vi "svfa_Initial Guess for Tone Estimation (magnitude).vi"(8 "FFT size":i32, 9 "window size":i32, 10 "window":T1(ring), 11 "three fingers":cluster{"f0":dbl, "df":dbl, "spectrum":dbl[]}={"f0"=0.0, "df"=1.0, "spectrum"=[]} {"spectrum" format="%.4f"; "df" format="%.4f"; "f0" format="%.4f"}) -> (0 "range":cluster{"f upper":dbl, "f lower":dbl} {"f lower" format="%.2e"; "f upper" format="%.2e"}, 3 "initial guess":dbl format="%.9f")   [LabVIEW 2017]
uses:
  <vilib>/Analysis/4window.llb/windowTd.ctl
  <vilib>/addons/_NISVFA/_Spectrum Processing/subVIs/svfa_Tone Estimation Subroutine G(f) (magnitude).vi
  <vilib>/addons/_NISVFA/_Spectrum Processing/subVIs/svfa_Tone Estimation Subroutine G(f) (first derivative) (magnitude).vi
  <vilib>/Analysis/NI_AALPro.lvlib
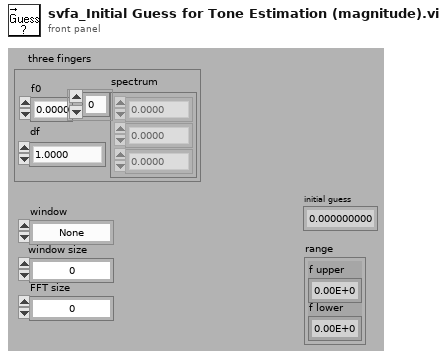
[diagram p1: front panel]
types:
  T1 = enum16{"None ", "Hanning", "Hamming", "Blackman-Harris", "Exact Blackman", "Blackman", "Flat Top", "4 Term B-Harris ", "7 Term B-Harris", "Low Sidelobe"}
  T2 = typedef "NI_AALPro.lvlib/windowTd.ctl" = u32
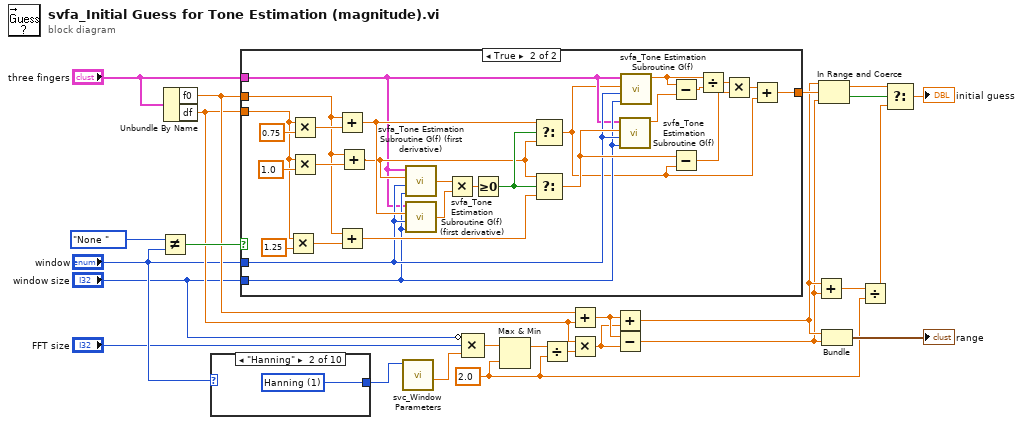
[diagram p0: block diagram]
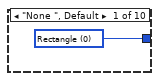
[diagram p2: hidden frame]
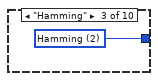
[diagram p3: hidden frame]
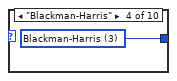
[diagram p4: hidden frame]
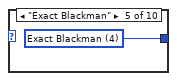
[diagram p5: hidden frame]
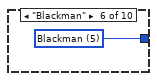
[diagram p6: hidden frame]
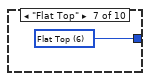
[diagram p7: hidden frame]
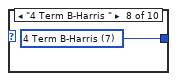
[diagram p8: hidden frame]
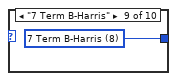
[diagram p9: hidden frame]
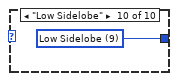
[diagram p10: hidden frame]
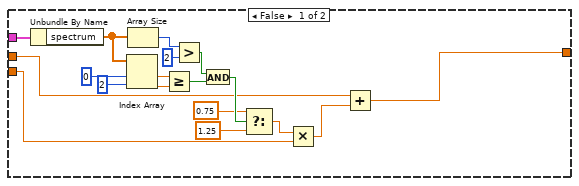
[diagram p11: hidden frame]
diagram:
  w3 = 2.0 ("y")
  n1 = Not Equal?(x=T1."None " ("window"), y="window") -> (x != y?=w23:bool)
  n2 = Unbundle By Name("three fingers") -> ("f0"=w17:dbl, "df"=w14:dbl)
  n3 = case shown="\"Hanning\"" "window" {
    tunnel: [w26 w27 w28 w29 w30 w31 w32 w33 w34 w35] -> w4
    frame "None ", Default {
      w26 = T2 0 items=["Rectangle"=0, "Hanning"=1, "Hamming"=2, "Blackman-Harris"=3, "Exact Blackman"=4, "Blackman"=5, "Flat Top"=6, "4 Term B-Harris "=7, "7 Term B-Harris"=8, "Low Sidelobe"=9, "Blackman Nuttall"=11, "Triangle"=30, "Bartlett-Hanning"=31, "Bohman"=32, "Parzen"=33, "Welch"=34, "Kaiser"=60, "Dolph-Chebyshev"=61, "Gaussian"=62] ("window")
    }
    frame "Hanning" {
      w27 = T2 1 items=["Rectangle"=0, "Hanning"=1, "Hamming"=2, "Blackman-Harris"=3, "Exact Blackman"=4, "Blackman"=5, "Flat Top"=6, "4 Term B-Harris "=7, "7 Term B-Harris"=8, "Low Sidelobe"=9, "Blackman Nuttall"=11, "Triangle"=30, "Bartlett-Hanning"=31, "Bohman"=32, "Parzen"=33, "Welch"=34, "Kaiser"=60, "Dolph-Chebyshev"=61, "Gaussian"=62] ("window")
    }
    frame "Hamming" {
      w28 = T2 2 items=["Rectangle"=0, "Hanning"=1, "Hamming"=2, "Blackman-Harris"=3, "Exact Blackman"=4, "Blackman"=5, "Flat Top"=6, "4 Term B-Harris "=7, "7 Term B-Harris"=8, "Low Sidelobe"=9, "Blackman Nuttall"=11, "Triangle"=30, "Bartlett-Hanning"=31, "Bohman"=32, "Parzen"=33, "Welch"=34, "Kaiser"=60, "Dolph-Chebyshev"=61, "Gaussian"=62] ("window")
    }
    frame "Blackman-Harris" {
      w29 = T2 3 items=["Rectangle"=0, "Hanning"=1, "Hamming"=2, "Blackman-Harris"=3, "Exact Blackman"=4, "Blackman"=5, "Flat Top"=6, "4 Term B-Harris "=7, "7 Term B-Harris"=8, "Low Sidelobe"=9, "Blackman Nuttall"=11, "Triangle"=30, "Bartlett-Hanning"=31, "Bohman"=32, "Parzen"=33, "Welch"=34, "Kaiser"=60, "Dolph-Chebyshev"=61, "Gaussian"=62] ("window")
    }
    frame "Exact Blackman" {
      w30 = T2 4 items=["Rectangle"=0, "Hanning"=1, "Hamming"=2, "Blackman-Harris"=3, "Exact Blackman"=4, "Blackman"=5, "Flat Top"=6, "4 Term B-Harris "=7, "7 Term B-Harris"=8, "Low Sidelobe"=9, "Blackman Nuttall"=11, "Triangle"=30, "Bartlett-Hanning"=31, "Bohman"=32, "Parzen"=33, "Welch"=34, "Kaiser"=60, "Dolph-Chebyshev"=61, "Gaussian"=62] ("window")
    }
    frame "Blackman" {
      w31 = T2 5 items=["Rectangle"=0, "Hanning"=1, "Hamming"=2, "Blackman-Harris"=3, "Exact Blackman"=4, "Blackman"=5, "Flat Top"=6, "4 Term B-Harris "=7, "7 Term B-Harris"=8, "Low Sidelobe"=9, "Blackman Nuttall"=11, "Triangle"=30, "Bartlett-Hanning"=31, "Bohman"=32, "Parzen"=33, "Welch"=34, "Kaiser"=60, "Dolph-Chebyshev"=61, "Gaussian"=62] ("window")
    }
    frame "Flat Top" {
      w32 = T2 6 items=["Rectangle"=0, "Hanning"=1, "Hamming"=2, "Blackman-Harris"=3, "Exact Blackman"=4, "Blackman"=5, "Flat Top"=6, "4 Term B-Harris "=7, "7 Term B-Harris"=8, "Low Sidelobe"=9, "Blackman Nuttall"=11, "Triangle"=30, "Bartlett-Hanning"=31, "Bohman"=32, "Parzen"=33, "Welch"=34, "Kaiser"=60, "Dolph-Chebyshev"=61, "Gaussian"=62] ("window")
    }
    frame "4 Term B-Harris " {
      w33 = T2 7 items=["Rectangle"=0, "Hanning"=1, "Hamming"=2, "Blackman-Harris"=3, "Exact Blackman"=4, "Blackman"=5, "Flat Top"=6, "4 Term B-Harris "=7, "7 Term B-Harris"=8, "Low Sidelobe"=9, "Blackman Nuttall"=11, "Triangle"=30, "Bartlett-Hanning"=31, "Bohman"=32, "Parzen"=33, "Welch"=34, "Kaiser"=60, "Dolph-Chebyshev"=61, "Gaussian"=62] ("window")
    }
    frame "7 Term B-Harris" {
      w34 = T2 8 items=["Rectangle"=0, "Hanning"=1, "Hamming"=2, "Blackman-Harris"=3, "Exact Blackman"=4, "Blackman"=5, "Flat Top"=6, "4 Term B-Harris "=7, "7 Term B-Harris"=8, "Low Sidelobe"=9, "Blackman Nuttall"=11, "Triangle"=30, "Bartlett-Hanning"=31, "Bohman"=32, "Parzen"=33, "Welch"=34, "Kaiser"=60, "Dolph-Chebyshev"=61, "Gaussian"=62] ("window")
    }
    frame "Low Sidelobe" {
      w35 = T2 9 items=["Rectangle"=0, "Hanning"=1, "Hamming"=2, "Blackman-Harris"=3, "Exact Blackman"=4, "Blackman"=5, "Flat Top"=6, "4 Term B-Harris "=7, "7 Term B-Harris"=8, "Low Sidelobe"=9, "Blackman Nuttall"=11, "Triangle"=30, "Bartlett-Hanning"=31, "Bohman"=32, "Parzen"=33, "Welch"=34, "Kaiser"=60, "Dolph-Chebyshev"=61, "Gaussian"=62] ("window")
    }
  }
  n4 = case shown="True" w23 {
    tunnel: [w52 w73] -> w25
    tunnel: "three fingers" -> [w41 w57]
    tunnel: w17 -> [w36 w54]
    tunnel: w14 -> [w37 w64]
    tunnel: "window" -> [_ w59]
    tunnel: "window size" -> [_ w58]
    frame False {
      n5 = Unbundle By Name(w41) -> ("spectrum"=w38:dbl[])
      n6 = Index Array(array=w38, index #1=0 ("Index"), index #2=2 ("Index")) -> (element #1=w40:dbl, element #2=w39:dbl)
      n7 = Array Size(array=w38) -> (size(s)=w46:i32)
      n8 = Greater Or Equal?(x=w40, y=w39) -> (x >= y?=w49:bool)
      n9 = Greater?(x=w46, y=2) -> (0:w44:bool)
      n10 = And(x=w44, y=w49) -> (x .and. y?=w47:bool)
      n11 = Select(t=0.75 ("x"), s=w47, f=1.25) -> (s? t:f=w48:dbl)
      n12 = Multiply(x=w48, y=w37) -> (x*y=w53:dbl)
      n13 = Add(x=w36, y=w53) -> (x+y=w52:dbl)
    }
    frame True {
      n14 = Multiply(x=w64, y=1.25 ("f")) -> (x*y=w68:dbl)
      n15 = Multiply(x=w64, y=0.75 ("t")) -> (x*y=w79:dbl)
      n16 = Multiply(x=w64, y=1.0 ("f")) -> (x*y=w78:dbl)
      n17 = Add(x=w54, y=w79) -> (x+y=w61:dbl)
      n18 = Add(x=w54, y=w68) -> (x+y=w62:dbl)
      n19 = Add(x=w54, y=w78) -> (x+y=w60:dbl)
      n20 = call-poly <vilib>:"svfa_Tone Estimation Subroutine G(f) (first derivative).vi"("N (window length)"=w58, "window"=w59, "frequency"=w60, "three fingers"=w57) -> ("G'(f)"=w56:dbl)
      n21 = call-poly <vilib>:"svfa_Tone Estimation Subroutine G(f) (first derivative).vi"("N (window length)"=w58, "window"=w59, "frequency"=w61, "three fingers"=w57) -> ("G'(f)"=w63:dbl)
      n22 = Multiply(x=w56, y=w63) -> (x*y=w67:dbl)
      n23 = Greater Or Equal To 0?(x=w67) -> (x >= 0?=w66:bool)
      n24 = Select(t=w61, s=w66, f=w60) -> (s? t:f=w55:dbl)
      n25 = Select(t=w60, s=w66, f=w62) -> (s? t:f=w65:dbl)
      n26 = call-poly <vilib>:"svfa_Tone Estimation Subroutine G(f).vi"("N (window length)"=w58, "window"=w59, "frequency"=w65, "three fingers"=w57) -> ("G(f)"=w76:dbl)  [unwired: 2 in, 1 out]
      n27 = call-poly <vilib>:"svfa_Tone Estimation Subroutine G(f).vi"("N (window length)"=w58, "window"=w59, "frequency"=w55, "three fingers"=w57) -> ("G(f)"=w72:dbl)  [unwired: 2 in, 1 out]
      n28 = Subtract(x=w72, y=w76) -> (x-y=w77:dbl)
      n29 = Subtract(x=w65, y=w55) -> (x-y=w71:dbl)
      n30 = Divide(x=w72, y=w77) -> (x/y=w75:dbl)
      n31 = Multiply(x=w75, y=w71) -> (x*y=w74:dbl)
      n32 = Add(x=w74, y=w55) -> (x+y=w73:dbl)
    }
  }
  n33 = call <vilib>:"svc_Window Parameters.vi"("window"=w4) -> ("6dB BW"=w6:dbl)  [unwired: 7 in, 3 out]
  n34 = Compound Arithmetic op=MULTIPLY(invert "window size", "FFT size", w6) -> (w16:dbl)
  n35 = Max & Min(x=w16, y=w3) -> (max(x,y)=w20:dbl)  [unwired: 1 out]
  n36 = Divide(x=w20, y=w3) -> (x/y=w21:dbl)
  n37 = Add(x=w17, y=w14) -> (x+y=w22:dbl)
  n38 = Multiply(x=w14, y=w21) -> (x*y=w15:dbl)
  n39 = Add(x=w22, y=w15) -> (x+y=w10:dbl)
  n40 = Subtract(x=w22, y=w15) -> (x-y=w9:dbl)
  n41 = Add(x=w10, y=w9) -> (x+y=w8:dbl)
  n42 = In Range and Coerce(upper limit=w10, x=w25, lower limit=w9) -> (coerced(x)=w13:dbl, In Range?=w11:bool)
  n43 = Bundle(w10, w9) -> (→"range":cluster{dbl, dbl})  [unwired: 1 in]
  n44 = Divide(x=w8, y=w3) -> (x/y=w7:dbl)
  n45 = Select(t=w13, s=w11, f=w7) -> (s? t:f=→"initial guess":dbl)
